vi "Start Async.vi"(8 "error in (no error)":errorcluster, 11 "gRPC service in":refnum<class "PluginLoader.lvclass">) -> (0 "error out":errorcluster, 3 "gRPC service out":refnum<class "PluginLoader.lvclass">)   [LabVIEW 2021, in "CIF_PluginLoader_server.lvlib" / "PluginLoader.lvclass"]
uses:
  PluginLoader.lvclass
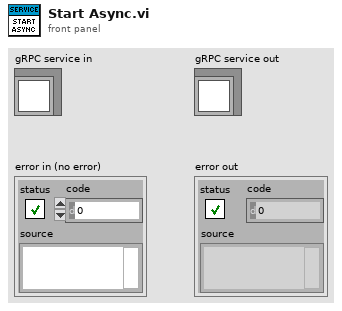
[diagram p1: front panel]
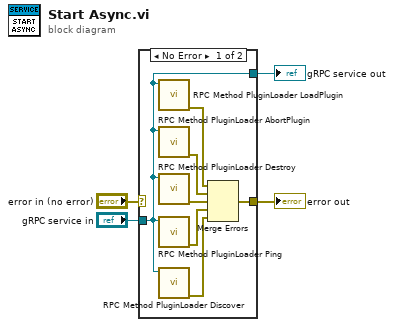
[diagram p0: block diagram]
diagram:
  n1 = case shown="No Error" "error in (no error)" {
    selector: "error in (no error)" -> [_ w13]
    tunnel: [w11 w13] -> w3
    tunnel: [w10 w12] -> w1
    tunnel: "gRPC service in" -> [w10 w12]
    frame No Error {
      n2 = call "RPC Method PluginLoader LoadPlugin.vi"("gRPC service in"=w10) -> ("error out"=w9:errorcluster)  [unwired: 9 in, 1 out]
      n3 = call "RPC Method PluginLoader AbortPlugin.vi"("gRPC service in"=w10) -> ("error out"=w8:errorcluster)  [unwired: 9 in, 1 out]
      n4 = call "RPC Method PluginLoader Destroy.vi"("gRPC service in"=w10) -> ("error out"=w7:errorcluster)  [unwired: 9 in, 1 out]
      n5 = call "RPC Method PluginLoader Ping.vi"("gRPC service in"=w10) -> ("error out"=w6:errorcluster)  [unwired: 9 in, 1 out]
      n6 = call "RPC Method PluginLoader Discover.vi"("gRPC service in"=w10) -> ("error out"=w5:errorcluster)  [unwired: 9 in, 1 out]
      n7 = Merge Errors(w9, w8, w7, w6, w5) -> (w11:errorcluster)
    }
    frame Error {
    }
  }
  "error out" <- w3
  "gRPC service out" <- w1
